vi "Source tag - explicit.vi"(8 "error in (no error)":errorcluster) -> (0 "error out":errorcluster)   [LabVIEW 2026, in "Tests.lvlib"]
doc: "Integration test (Caraya). Verifies a statement logged through the Logger reaches a single registered appender. Launches a manager with the default file disabled and a queue-mode relay capture probe (Open Test Mgr), logs one INFO statement, dequeues from the capture queue with a timeout, and asserts it was delivered and its message matches. Tears down with Close Test Mgr regardless of assertion outcome (SRS-LMBR-019). Uses the manager fixture; no temp root needed.\n\nImplements LMBR-T-019 -> SRS-013. Assert-level IDs: Test-ID-Assert-Checklist.md."
uses:
  Tests.lvlib
  src/TypeDefs/Severity.ctl
  <vilib>/addons/_JKI Toolkits/Caraya/classes/Assert/Assert Equal Value_Variant.vi
  <vilib>/addons/_JKI Toolkits/Caraya/classes/Test/Test.lvclass
  src/Lumberjack.lvlib
  src/Public/Logger.lvclass/Logger.lvclass
  <vilib>/addons/_JKI Toolkits/Caraya/classes/Assert/Assert.lvclass
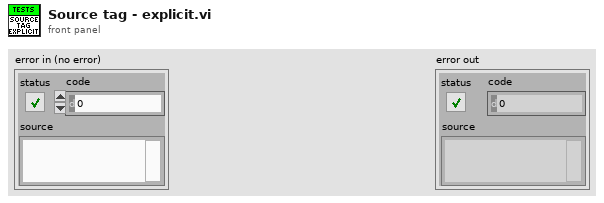
[diagram p1: front panel]
types:
  T1 = typedef "Lumberjack.lvlib/Severity.ctl" = enum16{"OFF", "FATAL", "ERROR", "WARN", "INFO", "DEBUG", "TRACE", "ALL"}
  T2 = typedef "Lumberjack.lvlib/Statement.ctl" = cluster{"timestamp":timestamp, "level":T1, "sourceTag":string, "originVI":string, "message":string}
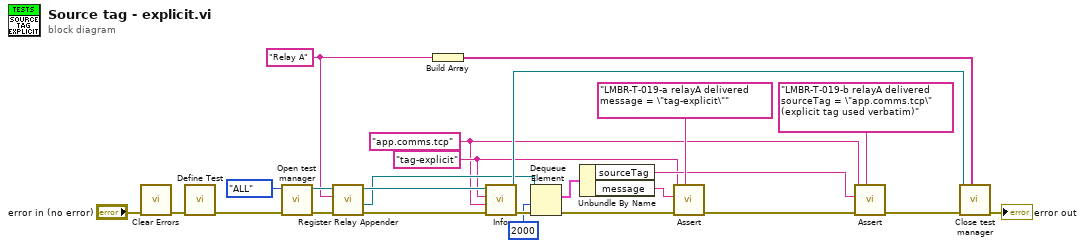
[diagram p0: block diagram]
diagram:
  w3 = "app.comms.tcp" ("sourceTag")
  w12 = "Relay A" ("id in")
  w4 = "tag-explicit" ("message")
  n1 = call <vilib>:"Clear Errors.vi"("error in (no error)"="error in (no error)") -> ("error out"=w1:errorcluster)  [unwired: 5 in, 1 out]
  n2 = call <vilib>:"Define Test.vi"("error in (no error)"=w1) -> ("error out"=w25:errorcluster)  [unwired: 9 in, 1 out]
  n3 = call "Open test manager.vi"("error in (no error)"=w25, "globalThreshold"=Severity."ALL") -> ("error out"=w16:errorcluster, "Logger out"=w17:refnum<class "Logger.lvclass">)  [unwired: 8 in]
  n4 = call "Register Relay Appender.vi"("error in (no error)"=w16, "id in"=w12, "Logger in"=w17) -> ("error out"=w14:errorcluster, "relayQueue"=w13:refnum<queue>, "Logger out"=w15:refnum<class "Logger.lvclass">)  [unwired: 5 in, 1 out]
  n5 = Build Array(w12) -> (w10:string[])
  n6 = call "Info.vi"("error in (no error)"=w14, "sourceTag"=w3, "message"=w4, "Logger in"=w15) -> ("error out"=w23:errorcluster, "Logger out"=w19:refnum<class "Logger.lvclass">)  [unwired: 6 in]
  n7 = Dequeue Element(queue=w13, timeout in ms (-1)=2000, error in (no error)=w23) -> (element=w21:T2, error out=w9:errorcluster)  [unwired: 2 out]
  n8 = Unbundle By Name(w21) -> ("sourceTag"=w5:string, "message"=w20:string)
  n9 = call-poly <vilib>:"Assert.vi"("Label"="LMBR-T-019-a relayA delivered message = \"tag-explicit\"", "error in (no error)"=w9, "Actual"=w20, "Expected"=w4) -> ("error out"=w7:errorcluster)  [unwired: 6 in, 1 out]
  n10 = call-poly <vilib>:"Assert.vi"("Label"="LMBR-T-019-b relayA delivered sourceTag = \"app.comms.tcp\" (explicit tag used verbatim)", "error in (no error)"=w7, "Actual"=w5, "Expected"=w3) -> ("error out"=w6:errorcluster)  [unwired: 6 in, 1 out]
  n11 = call "Close test manager.vi"("queueIDList"=w10, "error in (no error)"=w6, "Logger in"=w19) -> ("error out"=→"error out":errorcluster)  [unwired: 6 in]
